vi "Set Coil Constant.vi"(2 "error in":T1, 3 "Coil Constant (kG/A)":dbl format="%.5f", 4 "VISA resource name":refnum<visa-resource-name>) -> (0 "error out":T1, 1 "VISA resource name out":refnum<visa-resource-name>)   [LabVIEW 2019]
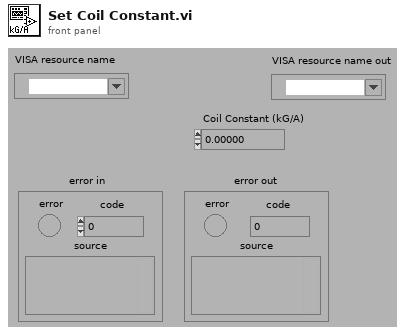
[diagram p1: front panel]
types:
  T1 = cluster{"error":bool, "code":i32, "source":string}
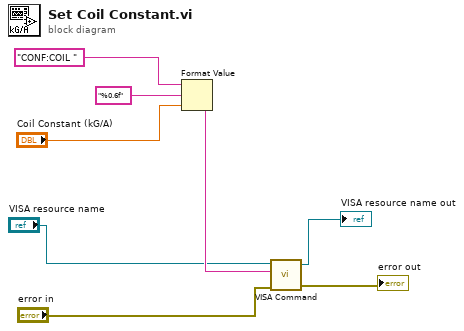
[diagram p0: block diagram]
diagram:
  n1 = Format Value(string ("")="CONF:COIL ", format string="%0.6f", value (0)="Coil Constant (kG/A)") -> (output string=w5:string)
  n2 = call "VISA Command.vi"("error in (no error)"="error in", "Command"=w5, "VISA resource name"="VISA resource name") -> ("error out"=→"error out":errorcluster, "VISA resource name out"=→"VISA resource name out":refnum<visa-resource-name>)  [unwired: 1 in, 1 out]
